vi "FdxGetErrorDescription.vi"(8 "error in":errorcluster, 11 "fdx_error_code":i32) -> (0 "error out":errorcluster, 3 "string description":string)   [LabVIEW 2020, in "AIM664LV.lvlib"]
uses:
  AIM664LV.lvlib
  FdxGlobalDllPath.vi
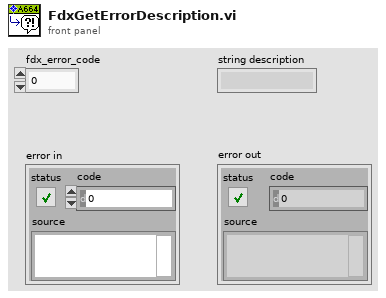
[diagram p1: front panel]
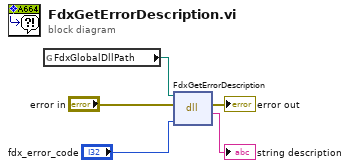
[diagram p0: block diagram]
diagram:
  n1 = global read "FdxGlobalDllPath.vi" "FdxGlobalDllPath"() -> (w1:path)
  n2 = dll-call lib="aim_fdx.19.dll" fn="FdxGetErrorDescription"(path in=w1, error in="error in", "fdx_error_code"="fdx_error_code") -> (error out=→"error out":errorcluster, "string description"=→"string description":string)  [unwired: 2 in, 1 out]
